vi "Set Joint Efforts.vi"(8 "error in (no error)":errorcluster, 10 "joint_efforts":dbl[](array[numeric]), 11 "GripsMaster in":refnum<class "GripsMaster.lvclass">) -> (0 "error out":errorcluster, 3 "GripsMaster out":refnum<class "GripsMaster.lvclass">)   [LabVIEW 2011, in "GripsMaster.lvclass"]
uses:
  GripsMaster.lvclass
  GripsMaster.lvclass/GripsMaster.ctl
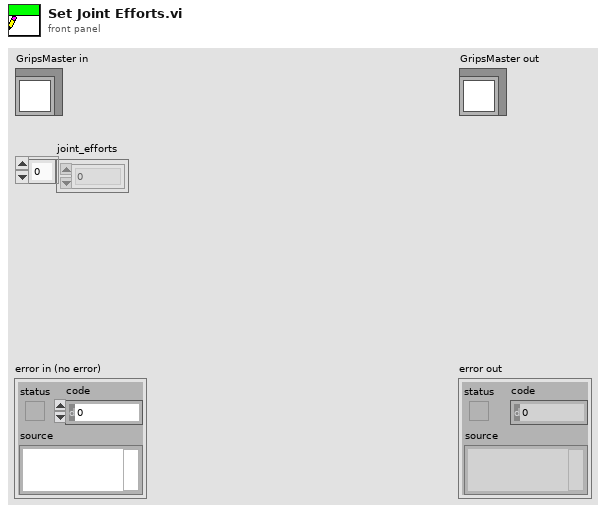
[diagram p1: front panel]
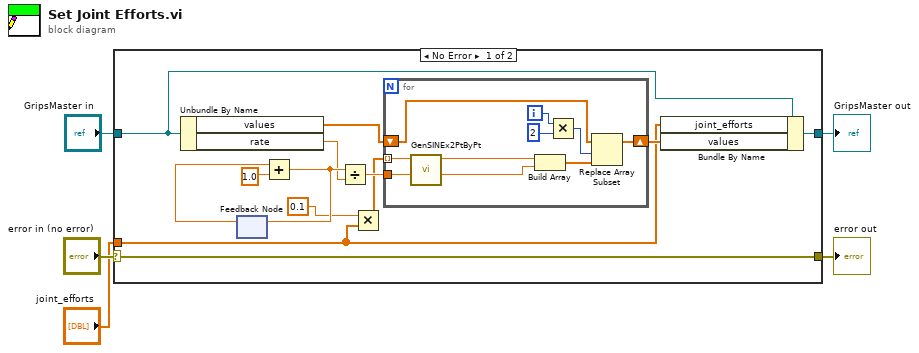
[diagram p0: block diagram]
diagram:
  n1 = case shown="No Error" "error in (no error)" {
    selector: "error in (no error)" -> [w18 w29]
    tunnel: [w18 w29] -> w4
    tunnel: [w17 w30] -> w2
    tunnel: "GripsMaster in" -> [w16 w30]
    tunnel: "joint_efforts" -> [w8 _]
    frame No Error {
      n2 = Unbundle By Name(w16) -> ("values"=w12:dbl[], "rate"=w9:dbl)
      n3 = feedback #1() -> (w14:dbl)  [unwired: 1 in]
      n4 = Add(x=w14, y=1.0 ("x")) -> (x+y=w13:dbl)
      n5 = feedback-in #1(w13) -> ()
      n6 = Divide(x=w13, y=w9) -> (x/y=w11:dbl)
      n7 = Multiply(x=0.1, y=w8) -> (x*y=w7:dbl[])
      n8 = for {
        shift-right: [w19] -> w10
        shift-left: w12 -> [w23]
        tunnel: w7 -> [w28] mode=indexing
        tunnel: w11 -> [w27]
        i -> [w26]
        n9 = call "GenSINEx2PtByPt.vi"("Time"=w27, "Acción de Control"=w28) -> ("Fase Control"=w21:dbl, "Fase Fija"=w22:dbl)  [unwired: 8 in]
        n10 = Build Array(w22, w21) -> (w20:dbl[])
        n11 = Multiply(x=w26, y=2) -> (x*y=w24:i32)
        n12 = Replace Array Subset(array=w23, new element=w20, index=w24) -> (w19:dbl[])
      }
      n13 = Bundle By Name(cluster=w16, "joint_efforts"=w8, "values"=w10) -> (w17:refnum<class "GripsMaster.lvclass">)
    }
    frame Error {
    }
  }
  "error out" <- w4
  "GripsMaster out" <- w2
